vi "Get Minimum Image Length.vi"(8 "error in (no error)":errorcluster, 11 "MinImageLength":i32) -> (0 "error out":errorcluster, 2 "function return":u32, 3 "MinImageLength out":i32)   [LabVIEW 2014, in "atmcd32d.lvlib"]
doc: "unsigned int WINAPI GetMinimumImageLength(int * MinImageLength);"
uses:
  atmcd32d.lvlib
  atmcd32d.dll
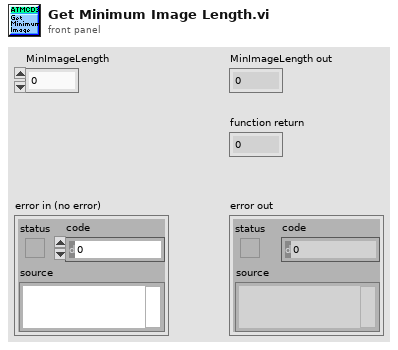
[diagram p1: front panel]
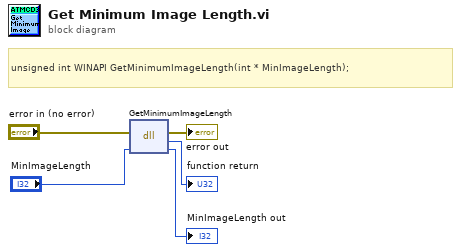
[diagram p0: block diagram]
diagram:
  # "unsigned int WINAPI GetMinimumImageLength(int * MinImageLength);"
  n1 = dll-call lib="C:/Users/Bakir/Documents/Lambda2-Testing/lib/Andorlib/atmcd32d.*" fn="GetMinimumImageLength"(error in="error in (no error)", "MinImageLength"="MinImageLength") -> (error out=→"error out":errorcluster, →"function return":u32, "MinImageLength"=→"MinImageLength out":i32)  [unwired: 2 in, 1 out]
